vi "KepcoDCPwr Configure Current Protect Level.vi"(0 "VISA Session":refnum<visa-resource-name>, 5 "Model In":string, 7 "channel name (\"\")":string="\"\"", 9 "level (0.0 volts)":dbl caption="level" format="%^.2e", 11 "error in (no error)":errorcluster {"code" format="%.0x"}) -> (4 "VISA Session Out":refnum<visa-resource-name>, 6 "Model Out":string, 8 "channel name out (\"\")":string="\"\"" caption="channel name Out (\"\")", 15 "error out":errorcluster {"code" format="%.0x"})   [LabVIEW 2020]
doc: "This VI configures the DC voltage level the power supply attempts to generate."
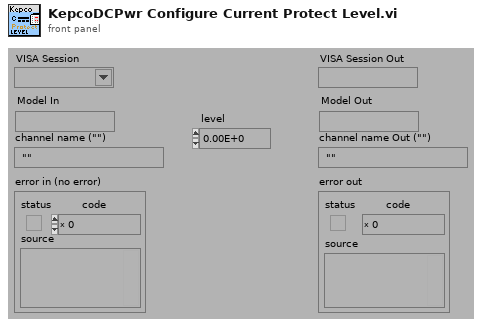
[diagram p1: front panel]
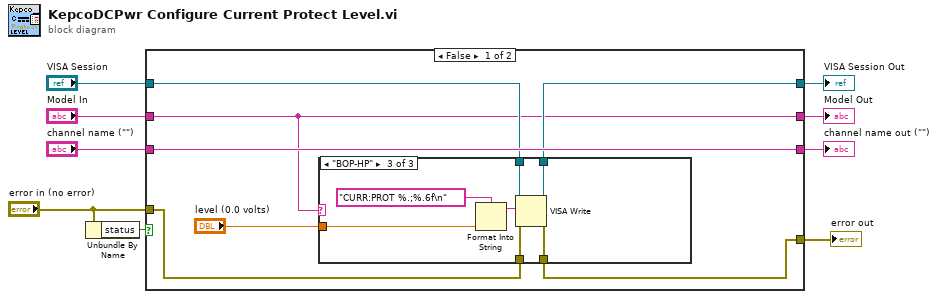
[diagram p0: block diagram]
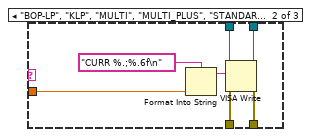
[diagram p3: hidden frame]
diagram:
  n1 = Unbundle By Name("error in (no error)") -> ("status"=w8:bool)
  n2 = case shown="False" w8 {
    tunnel: [w10 w36] -> w9
    tunnel: "error in (no error)" -> [w15 w36]
    tunnel: [w13 w35] -> w6
    tunnel: "VISA Session" -> [w14 w35]
    tunnel: "Model In" -> [w11 w34]
    tunnel: "channel name (\"\")" -> [w16 w33]
    tunnel: [w11 w34] -> w2
    tunnel: [w16 w33] -> w1
    frame False {
      n3 = case shown="\"BOP-HP\"" w11 {
        tunnel: w15 -> [w18 w25 w32]
        tunnel: [w18 w24 w31] -> w10
        tunnel: w14 -> [w17 w23 w30]
        tunnel: [w17 w22 w29] -> w13
        tunnel: "level (0.0 volts)" -> [_ w21 w28]
        frame "", Default {
        }
        frame "BOP-LP", "KLP", "MULTI", "MULTI_PLUS", "STANDARD" {
          n4 = Format Into String(format string="CURR %.;%.6f\n", w21) -> (resulting string=w19:string)  [unwired: 2 in, 1 out]
          n5 = VISA Write(VISA resource name=w23, write buffer=w19, error in (no error)=w25) -> (VISA resource name out=w22:refnum<visa-resource-name>, error out=w24:errorcluster)  [unwired: 1 out]
        }
        frame "BOP-HP" {
          n6 = Format Into String(format string="CURR:PROT %.;%.6f\n", w28) -> (resulting string=w26:string)  [unwired: 2 in, 1 out]
          n7 = VISA Write(VISA resource name=w30, write buffer=w26, error in (no error)=w32) -> (VISA resource name out=w29:refnum<visa-resource-name>, error out=w31:errorcluster)  [unwired: 1 out]
        }
      }
    }
    frame True {
    }
  }
  "error out" <- w9
  "VISA Session Out" <- w6
  "channel name out (\"\")" <- w1
  "Model Out" <- w2
